vi "CompleteMetadataRegistration.vi"(8 "error in":errorcluster, 11 "gRPC ID in":T1) -> (0 "error out":errorcluster, 3 "gRPC ID Out":T1)   [LabVIEW 2019, in "grpc-lvsupport.lvlib"]
uses:
  grpc-lvsupport.lvlib
  grpcId.ctl
  <vilib>/Utility/error.llb/Error Cluster From Error Code.vi
  <resource>/labview_grpc_server.dll
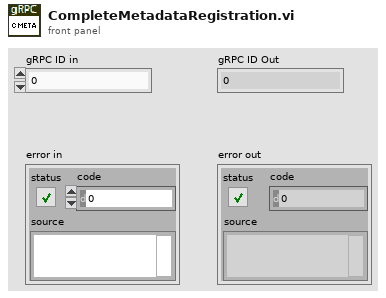
[diagram p1: front panel]
types:
  T1 = typedef "grpc-lvsupport.lvlib/grpcId.ctl" = u64
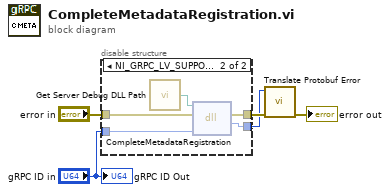
[diagram p0: block diagram]
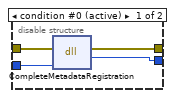
[diagram p2: hidden frame]
diagram:
  n1 = disable-structure shown="NI_GRPC_LV_SUPPORT_DEBUG==True&&RUN_TIME_ENGINE==False" {
    disable-tunnel: "error in" -> [w9 w14]
    disable-tunnel: [w8 w13] -> w4
    disable-tunnel: "gRPC ID in" -> [w7 w11]
    disable-tunnel: [w6 w10] -> w1
    frame condition #0 (active) {
      n2 = dll-call lib="C:/Program Files (x86)/National Instruments/LabVIEW 2024/resource/labview_grpc_server.*" fn="CompleteMetadataRegistration"(error in=w9, "serializationId"=w7) -> (error out=w8:errorcluster, "return type"=w6:i32)  [unwired: 3 in, 1 out]
    }
    frame condition #1 {
      n3 = call "Get Server Debug DLL Path.vi"() -> ("DLL Path"=w12:path)
      n4 = dll-call lib="?" fn="CompleteMetadataRegistration"(path in=w12, error in=w14, "serializationId"=w11) -> (error out=w13:errorcluster, "return type"=w10:i32)  [unwired: 2 in, 1 out]
    }
  }
  n5 = call "Translate Protobuf Error.vi"("error in"=w4, "Error Code"=w1) -> ("error out"=→"error out":errorcluster)  [unwired: 9 in]
  "gRPC ID Out" <- "gRPC ID in"
